vi "Get Wire Next Element.vi"(11 "wire in":refnum<vi>) -> (2 "next terminal datatype":string, 3 "next terminal":refnum<vi>)   [LabVIEW 2014]
doc: "Returns next element on another end of wire and its datatype. It's used to traverse error wire, because error wire determines execution order."
panel:
  out "wire label":string
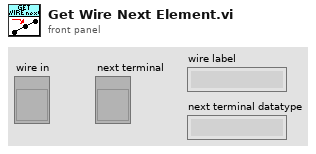
[diagram p1: front panel]
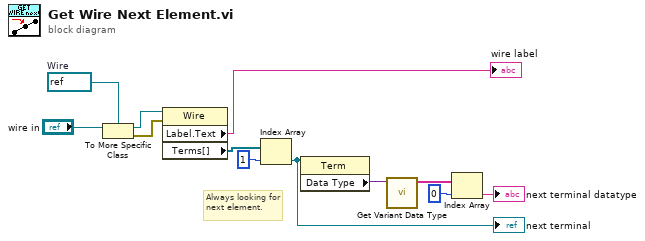
[diagram p0: block diagram]
diagram:
  w2 = refnum<vi> refnum  # Wire
  # "Always looking for next element."
  n1 = To More Specific Class(target class=w2, reference="wire in") -> (specific class reference=w10:refnum<vi>, error out=w3:errorcluster)  [unwired: 1 in]
  n2 = property on="Property Node" class="Wire"(reference=w10, error in=w3) -> ("Label.Text"=→"wire label":string, "Terms[]"=w4:refnum<vi>[])  [unwired: 2 out]
  n3 = Index Array(array=w4, index=1) -> (element=w11:refnum<vi>)
  "next terminal" <- w11
  n4 = property on="Property Node" class="Term"(reference=w11) -> ("Data Type"=w5:variant)  [unwired: 1 in, 2 out]
  n5 = call "Get Variant Data Type.vi"("variant"=w5) -> ("Data Type"=w6:string[])  [unwired: 10 in]
  n6 = Index Array(array=w6, index=0) -> (element=→"next terminal datatype":string)
